vi "_histUpdate.vi"(9 "Y:0-U:1-R:2":i32, 10 "History In":dbl[][][](array[numeric]), 11 "pry":dbl[](array[numeric])) -> (2 "History Out":dbl[][][](array[numeric]))   [LabVIEW 2021, in "System.lvclass"]
uses:
  System.lvclass
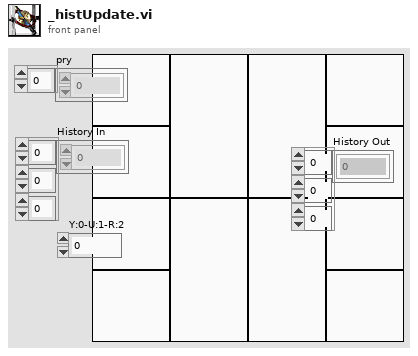
[diagram p1: front panel]
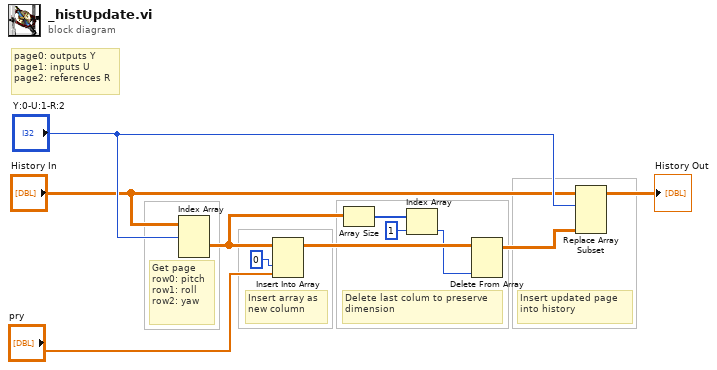
[diagram p0: block diagram]
diagram:
  # "Insert updated page into history"
  # "Delete last colum to preserve dimension"
  # "Insert array as new column"
  # "Get page\nrow0: pitch\nrow1: roll\nrow2: yaw"
  # "page0: outputs Y\npage1: inputs U\npage2: references R"
  n1 = Index Array(array="History In", index (dim 0)="Y:0-U:1-R:2") -> (element=w9:dbl[][])  [unwired: 2 in]
  n2 = Insert Into Array(array=w9, index (col)=0 ("disabled index (col)"), new element="pry") -> (w7:dbl[][])  [unwired: 1 in]
  n3 = Array Size(array=w9) -> (size(s)=w10:i32[])
  n4 = Index Array(array=w10, index=1) -> (element=w6:i32)
  n5 = Delete From Array(array=w7, index (col)=w6) -> (array with subset deleted=w5:dbl[][])  [unwired: 2 in, 1 out]
  n6 = Replace Array Subset(array="History In", new element=w5, index (dim 0)="Y:0-U:1-R:2") -> (→"History Out":dbl[][][])  [unwired: 2 in]
